vi "Infect.vi"(8 "Error In":errorcluster, 11 "Selection List[]":refnum<vi>[](array[refnum])) -> (0 "Error Out":errorcluster, 3 "Change Made?":bool)   [LabVIEW 2017, in "Eulogy.lvlib"]
doc: "Changes a grave site (Diagram Disable structure) to the Corpse frame (legacy code) and enables it. The \"Corpse\" label is replaced with a \"Zombie\" label and a timestamp of when the legacy code was re-enabled. In other words, infect the corpse with a zombie virus to revive it."
uses:
  Eulogy.lvlib
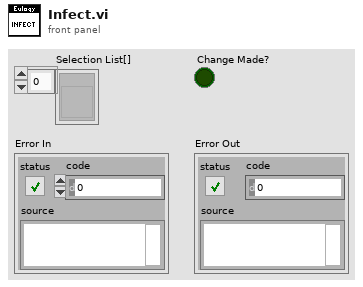
[diagram p1: front panel]
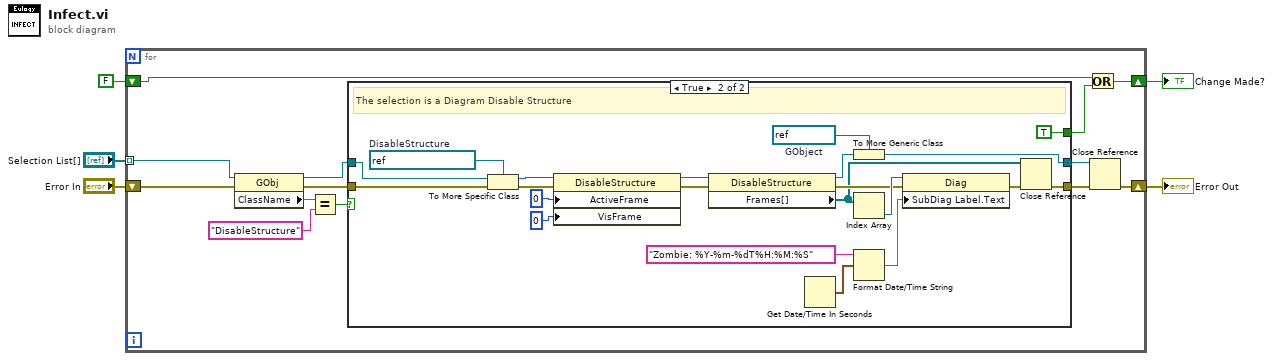
[diagram p0: block diagram]
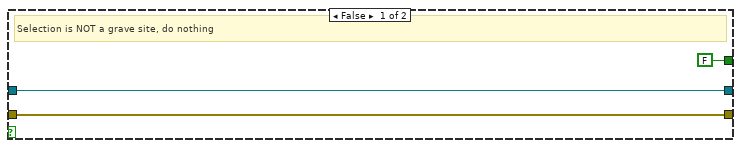
[diagram p2: hidden frame]
diagram:
  n1 = for {
    shift-right: [w6] -> w5
    shift-left: "Error In" -> [w18]
    tunnel: "Selection List[]" -> [w12] mode=indexing
    shift-right: [w9] -> w3
    shift-left: FALSE -> [w11]
    n2 = property class="GObj"(reference=w12, error in=w18) -> (reference out=w14:refnum<vi>, error out=w13:errorcluster, "ClassName"=w17:string)
    n3 = Equal?(x=w17, y="DisableStructure") -> (x = y?=w15:bool)
    n4 = case shown="True" w15 {
      tunnel: w14 -> [w20 w41]
      tunnel: w13 -> [w19 w40]
      tunnel: [FALSE ("y") TRUE ("y")] -> w10
      tunnel: [w19 w25] -> w8
      tunnel: [w20 w23] -> w7
      frame False {
        # "Selection is NOT a grave site, do nothing"
      }
      frame True {
        w22 = refnum<vi> refnum  # GObject
        w42 = refnum<vi> refnum  # DisableStructure
        # "The selection is a Diagram Disable Structure"
        n5 = To More Specific Class(target class=w42, reference=w41, error in=w40) -> (specific class reference=w38:refnum<vi>, error out=w39:errorcluster)
        n6 = property class="DisableStructure"(reference=w38, error in=w39, "ActiveFrame"=i16 0 ("Active Frame"), "VisFrame"=u32 0 ("Visible Frame")) -> (reference out=w35:refnum<vi>, error out=w34:errorcluster)
        n7 = property class="DisableStructure"(reference=w35, error in=w34) -> (reference out=w24:refnum<vi>, error out=w32:errorcluster, "Frames[]"=w27:refnum<vi>[])
        n8 = Get Date/Time In Seconds() -> (seconds since 1Jan1904=w31:timestamp)
        n9 = To More Generic Class(target class=w22, reference=w24) -> (generic class reference=w23:refnum<vi>)
        n10 = Index Array(array=w27) -> (element=w33:refnum<vi>)  [unwired: 1 in]
        n11 = Format Date/Time String(time format string (%c)="Zombie: %Y-%m-%dT%H:%M:%S", seconds (now)=w31) -> (date/time string=w29:string)  [unwired: 1 in]
        n12 = property class="Diag"(reference=w33, error in=w32, "SubDiag Label.Text"=w29) -> (error out=w28:errorcluster)  [unwired: 1 out]
        n13 = Close Reference(reference=w27, error in (no error)=w28) -> (error out=w25:errorcluster)
      }
    }
    n14 = Or(x=w11, y=w10) -> (x .or. y?=w9:bool)
    n15 = Close Reference(reference=w7, error in (no error)=w8) -> (error out=w6:errorcluster)
  }
  "Error Out" <- w5
  "Change Made?" <- w3
